vi "initialize_arduinos_subVI 11-08-2017.vi"(10 "arduino 1-6 addresses":T2, 11 "arduinos on?":bool) -> (3 "arduino addresses out":T1)   [LabVIEW 2014]
uses:
  <vilib>/Instr/_visa.llb/VISA Configure Serial Port (Instr).vi
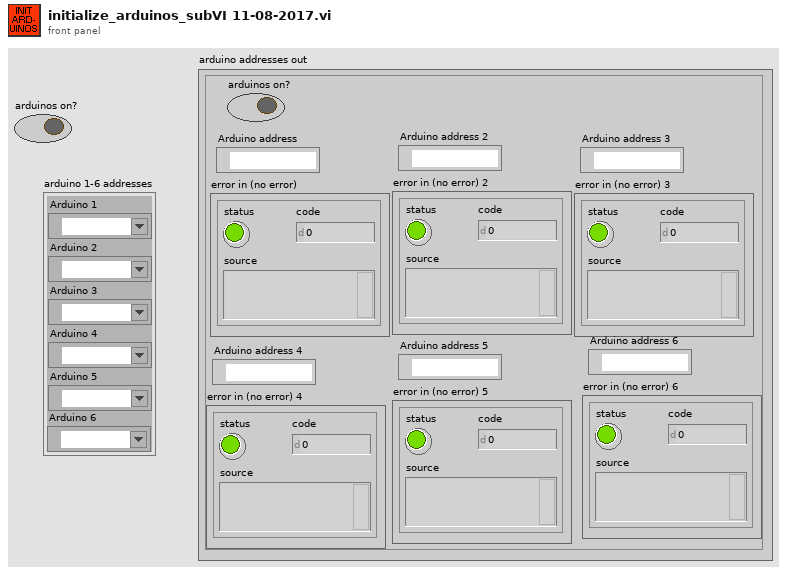
[diagram p1: front panel]
types:
  T1 = cluster{"Arduino address":refnum<visa-resource-name>, "error in (no error)":errorcluster, "Arduino address 2":refnum<visa-resource-name>, "error in (no error) 2":errorcluster, "Arduino address 3":refnum<visa-resource-name>, "error in (no error) 3":errorcluster, "Arduino address 4":refnum<visa-resource-name>, "error in (no error) 4":errorcluster, "Arduino address 5":refnum<visa-resource-name>, "error in (no error) 5":errorcluster, "Arduino address 6":refnum<visa-resource-name>, "error in (no error) 6":errorcluster, "arduinos on?":bool}
  T2 = cluster{"Arduino 1":refnum<visa-resource-name>, "Arduino 2":refnum<visa-resource-name>, "Arduino 3":refnum<visa-resource-name>, "Arduino 4":refnum<visa-resource-name>, "Arduino 5":refnum<visa-resource-name>, "Arduino 6":refnum<visa-resource-name>}
  T3 = cluster{"VISA resource name out":refnum<visa-resource-name>, "error out":errorcluster, "VISA resource name out":refnum<visa-resource-name>, "error out":errorcluster, "VISA resource name out":refnum<visa-resource-name>, "error out":errorcluster, "VISA resource name out":refnum<visa-resource-name>, "error out":errorcluster, "VISA resource name out":refnum<visa-resource-name>, "error out":errorcluster, "VISA resource name out":refnum<visa-resource-name>, "error out":errorcluster, bool}
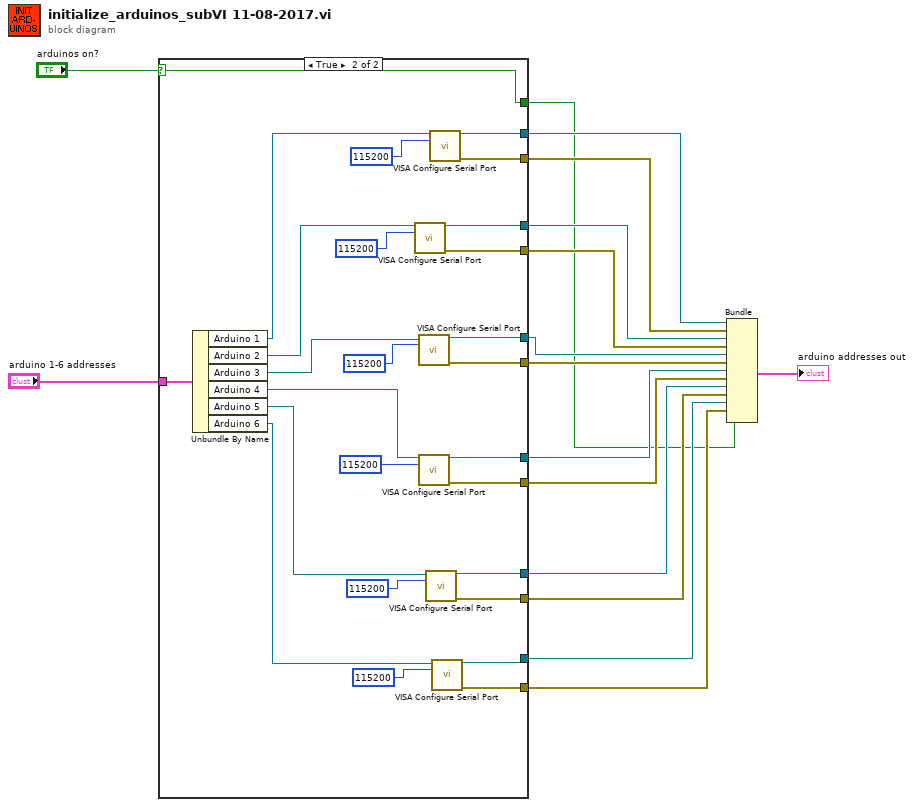
[diagram p0: block diagram]
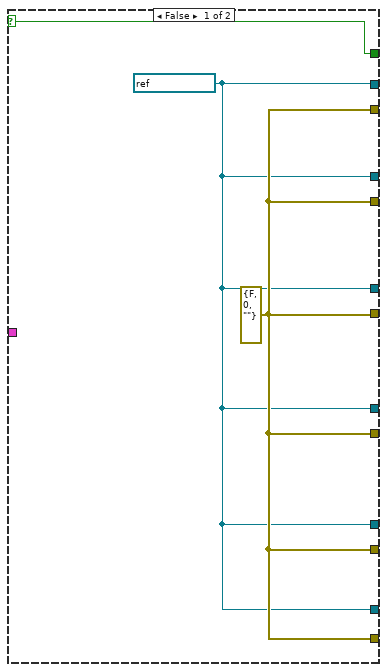
[diagram p2: hidden frame]
diagram:
  n1 = case shown="True" "arduinos on?" {
    selector: "arduinos on?" -> [w19 w45]
    tunnel: [w19 w45] -> w2
    tunnel: [w17 w43] -> w14
    tunnel: [w18 w42] -> w13
    tunnel: [w17 w40] -> w12
    tunnel: [w18 w39] -> w11
    tunnel: [w17 w37] -> w10
    tunnel: [w18 w36] -> w9
    tunnel: [w17 w33] -> w8
    tunnel: [w18 w32] -> w7
    tunnel: [w17 w31] -> w6
    tunnel: [w18 w30] -> w5
    tunnel: "arduino 1-6 addresses" -> [_ w26]
    tunnel: [w17 w28] -> w4
    tunnel: [w18 w27] -> w3
    frame False {
      w18 = errorcluster {"status"=FALSE, "code"=0, "source"=""} ("error out")
      w17 = refnum<visa-resource-name> refnum ("VISA resource name out")
    }
    frame True {
      n2 = Unbundle By Name(w26) -> ("Arduino 1"=w25:refnum<visa-resource-name>, "Arduino 2"=w24:refnum<visa-resource-name>, "Arduino 3"=w23:refnum<visa-resource-name>, "Arduino 4"=w22:refnum<visa-resource-name>, "Arduino 5"=w21:refnum<visa-resource-name>, "Arduino 6"=w20:refnum<visa-resource-name>)
      n3 = call-poly "VISA Configure Serial Port"("VISA resource name"=w24, "baud rate (9600)"=u32 115200) -> ("VISA resource name out"=w40:refnum<visa-resource-name>, "error out"=w39:errorcluster)  [unwired: 12 in]
      n4 = call-poly "VISA Configure Serial Port"("VISA resource name"=w23, "baud rate (9600)"=u32 115200) -> ("VISA resource name out"=w37:refnum<visa-resource-name>, "error out"=w36:errorcluster)  [unwired: 12 in]
      n5 = call-poly "VISA Configure Serial Port"("VISA resource name"=w22, "baud rate (9600)"=u32 115200) -> ("VISA resource name out"=w33:refnum<visa-resource-name>, "error out"=w32:errorcluster)  [unwired: 12 in]
      n6 = call-poly "VISA Configure Serial Port"("VISA resource name"=w21, "baud rate (9600)"=u32 115200) -> ("VISA resource name out"=w31:refnum<visa-resource-name>, "error out"=w30:errorcluster)  [unwired: 12 in]
      n7 = call-poly "VISA Configure Serial Port"("VISA resource name"=w25, "baud rate (9600)"=u32 115200) -> ("VISA resource name out"=w43:refnum<visa-resource-name>, "error out"=w42:errorcluster)  [unwired: 12 in]
      n8 = call-poly "VISA Configure Serial Port"("VISA resource name"=w20, "baud rate (9600)"=u32 115200) -> ("VISA resource name out"=w28:refnum<visa-resource-name>, "error out"=w27:errorcluster)  [unwired: 12 in]
    }
  }
  n9 = Bundle("VISA resource name out"=w14, "error out"=w13, "VISA resource name out"=w12, "error out"=w11, "VISA resource name out"=w10, "error out"=w9, "VISA resource name out"=w8, "error out"=w7, "VISA resource name out"=w6, "error out"=w5, "VISA resource name out"=w4, "error out"=w3, w2) -> (→"arduino addresses out":T3)  [unwired: 1 in]
